vi "DisconnectBase.vi"(8 "error in (no error)":errorcluster, 11 "Konvolucio MCAN120803 Adapter Class in":refnum<class "Konvolucio MCAN120803 Adapter Class.lvclass">) -> (0 "error out":errorcluster, 3 "Konvolucio MCAN120803 Adapter Class out":refnum<class "Konvolucio MCAN120803 Adapter Class.lvclass">)   [LabVIEW 2011, in "Konvolucio MCAN120803 Adapter Class.lvclass"]
uses:
  Konvolucio MCAN120803 Adapter Class.lvclass
  Generic CAN Adapter/GenericCanAdapterClass.lvclass
  Konvolucio MCAN120803 Adapter Class.lvclass/Konvolucio MCAN120803 Adapter Class.ctl
  <instrlib>/Konvolucio MCAN120803/Konvolucio MCAN120803.lvlib
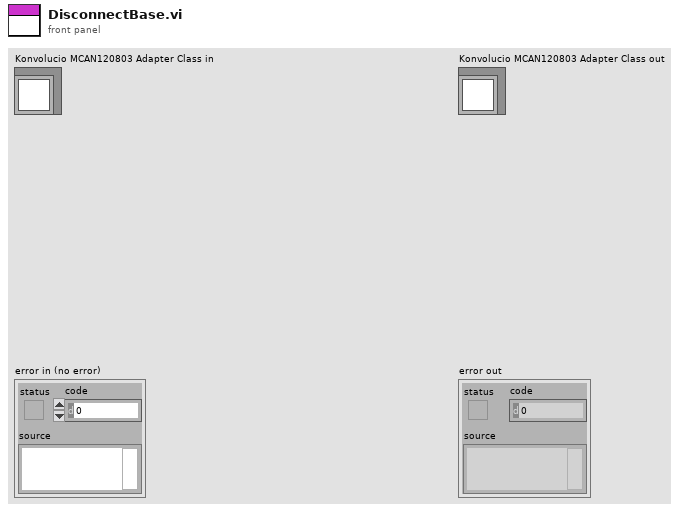
[diagram p1: front panel]
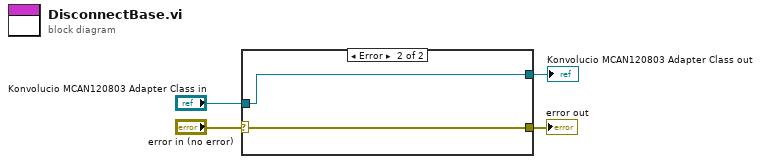
[diagram p0: block diagram]
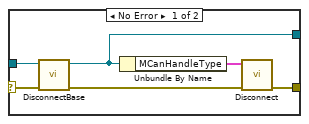
[diagram p2: hidden frame]
diagram:
  n1 = case shown="Error" "error in (no error)" {
    selector: "error in (no error)" -> [w5 w11]
    tunnel: "Konvolucio MCAN120803 Adapter Class in" -> [w10 w12]
    tunnel: [w9 w11] -> w3
    tunnel: [w7 w12] -> w2
    frame No Error {
      n2 = call-parent "DisconnectBase.vi"("error in (no error)"=w5, "GenericCanAdapterClass in"=w10) -> ("error out"=w8:errorcluster, "GenericCanAdapterClass out"=w7:refnum<class "Konvolucio MCAN120803 Adapter Class.lvclass">)  [unwired: 8 in]
      n3 = Unbundle By Name(w7) -> ("MCanHandleType"=w6:cluster{"MCanAdapter":refnum<k24>})
      n4 = call <instrlib>:"Disconnect.vi"("error in"=w8, "CanHandleIn"=w6) -> ("error out"=w9:errorcluster)  [unwired: 9 in]
    }
    frame Error {
    }
  }
  "error out" <- w3
  "Konvolucio MCAN120803 Adapter Class out" <- w2
